vi "VsEP-Find Next Level.vi"(0 "Runtime":T1, 11 "error in (no error)":errorcluster, 12 "Amplitude":dbl) -> (4 "Runtime out":T1, 14 "Finished":bool, 15 "error out":errorcluster)   [LabVIEW 2020]
uses:
  Typedefs/VsEP-Runtime Data.ctl
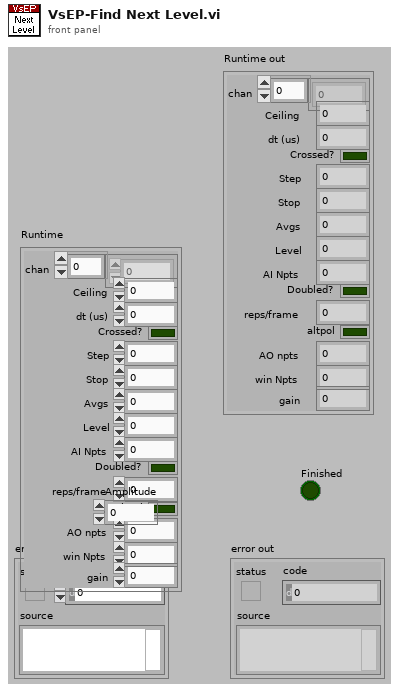
[diagram p1: front panel]
types:
  T1 = typedef "VsEP-Runtime Data.ctl" = cluster{"chan":i32[], "Ceiling":dbl, "dt (us)":dbl, "Crossed?":bool, "Step":dbl, "Stop":i32, "Avgs":i32, "Level":dbl, "AI Npts":i32, "Doubled?":bool, "reps/frame":i32, "altpol":bool, "AO npts":i32, "win Npts":i32, "gain":dbl}
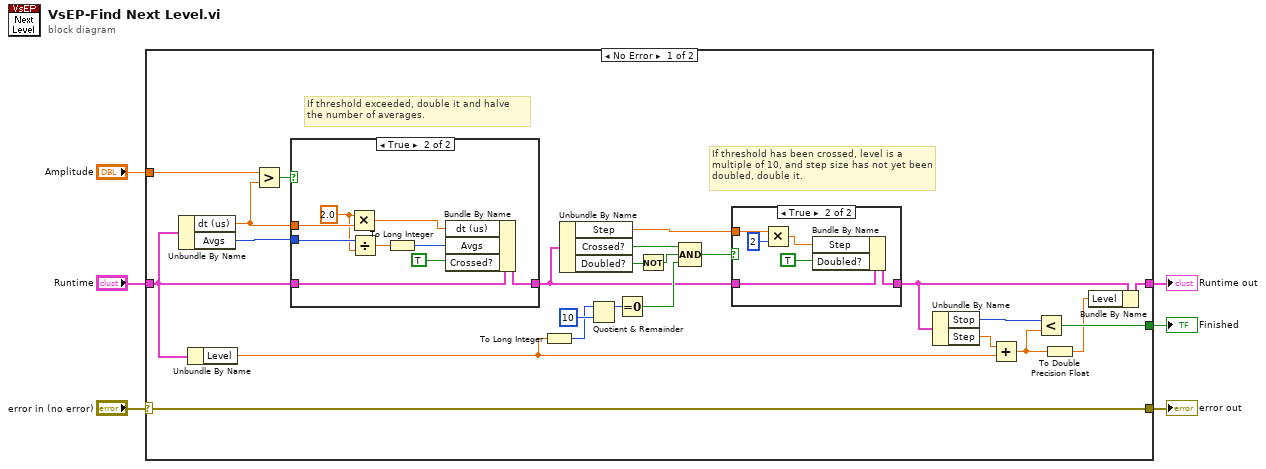
[diagram p0: block diagram]
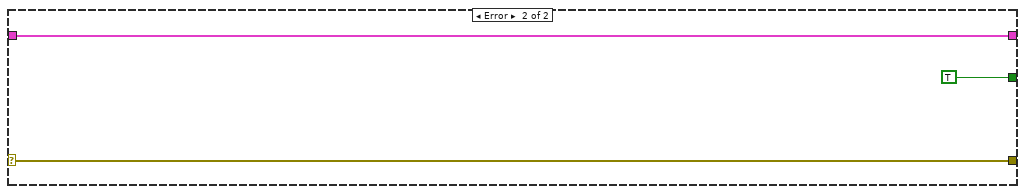
[diagram p4: hidden frame]
diagram:
  n1 = case shown="No Error" "error in (no error)" {
    selector: "error in (no error)" -> [w22 w49]
    tunnel: "Runtime" -> [w21 w50]
    tunnel: "Amplitude" -> [w30 _]
    tunnel: [w23 TRUE] -> w3
    tunnel: [w20 w50] -> w2
    tunnel: [w22 w49] -> w1
    frame No Error {
      # "If threshold has been crossed, level is a multiple of 10, and step size has not yet been doubled, double it."
      # "If threshold exceeded, double it and halve the number of averages."
      n2 = Unbundle By Name(w21) -> ("dt (us)"=w27:dbl, "Avgs"=w26:i32)
      n3 = Unbundle By Name(w21) -> ("Level"=w7:dbl)
      n4 = Greater?(x=w30, y=w27) -> (0:w18:bool)
      n5 = case shown="True" w18 {
        tunnel: w21 -> [w38 w40]
        tunnel: w27 -> [_ w47]
        tunnel: w26 -> [_ w46]
        tunnel: [w38 w42] -> w9
        frame False {
        }
        frame True {
          w45 = 2.0 ("y")
          n6 = Multiply(x=w45, y=w47) -> (x*y=w44:dbl)
          n7 = Divide(x=w46, y=w45) -> (x/y=w43:dbl)
          n8 = To Long Integer(number=w43) -> (32bit integer=w41:i32)
          n9 = Bundle By Name(cluster=w40, "dt (us)"=w44, "Avgs"=w41, "Crossed?"=TRUE) -> (w42:T1)
        }
      }
      n10 = To Long Integer(number=w7) -> (32bit integer=w16:i32)
      n11 = Unbundle By Name(w9) -> ("Step"=w10:dbl, "Crossed?"=w14:bool, "Doubled?"=w15:bool)
      n12 = Quotient & Remainder(x=w16, y=10) -> (x-y*floor(x/y)=w28:i32)  [unwired: 1 out]
      n13 = Equal To 0?(x=w28) -> (x = 0?=w12:bool)
      n14 = Not(x=w15) -> (.not. x?=w13:bool)
      n15 = Compound Arithmetic op=AND(w14, w13, w12) -> (w11:bool)
      n16 = case shown="True" w11 {
        tunnel: [w31 w34] -> w8
        tunnel: w10 -> [_ w33]
        tunnel: w9 -> [w31 w32]
        frame False {
        }
        frame True {
          n17 = Multiply(x=w33, y=2) -> (x*y=w36:dbl)
          n18 = Bundle By Name(cluster=w32, "Step"=w36, "Doubled?"=TRUE ("Crossed?")) -> (w34:T1)
        }
      }
      n19 = Unbundle By Name(w8) -> ("Stop"=w25:i32, "Step"=w17:dbl)
      n20 = Add(x=w17, y=w7) -> (x+y=w24:dbl)
      n21 = Less?(x=w25, y=w24) -> (x < y?=w23:bool)
      n22 = To Double Precision Float(number=w24) -> (double precision float=w19:dbl)
      n23 = Bundle By Name(cluster=w8, "Level"=w19) -> (w20:T1)
    }
    frame Error {
    }
  }
  "error out" <- w1
  "Runtime out" <- w2
  "Finished" <- w3
